vi "1lab11111.vi"() -> ()   [LabVIEW 2020]
panel:
  out "погрешность,%":dbl
  in  "шаг t":dbl
  out "Q":dbl(graph)
  in  "C эталонное":dbl
  out "Meter":dbl(knob) scale=0.0..10.0
  out "I":dbl(graph)
  out "U":dbl(graph)
  out "C. мкФ":dbl
  out "Величина заряда, мКл":dbl
  out "t разрядки":dbl
  in  "U конечное":dbl
  in  "U":dbl
  in  "R":dbl
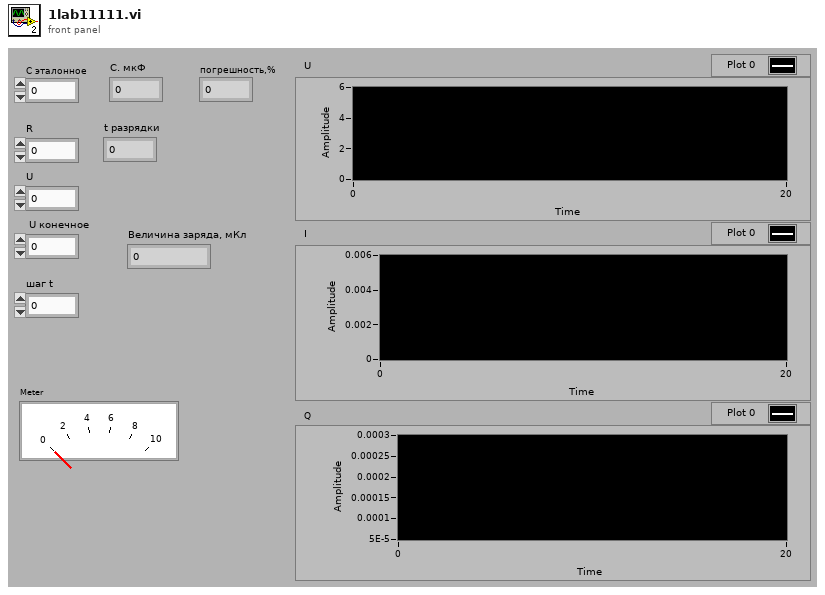
[diagram p1: front panel]
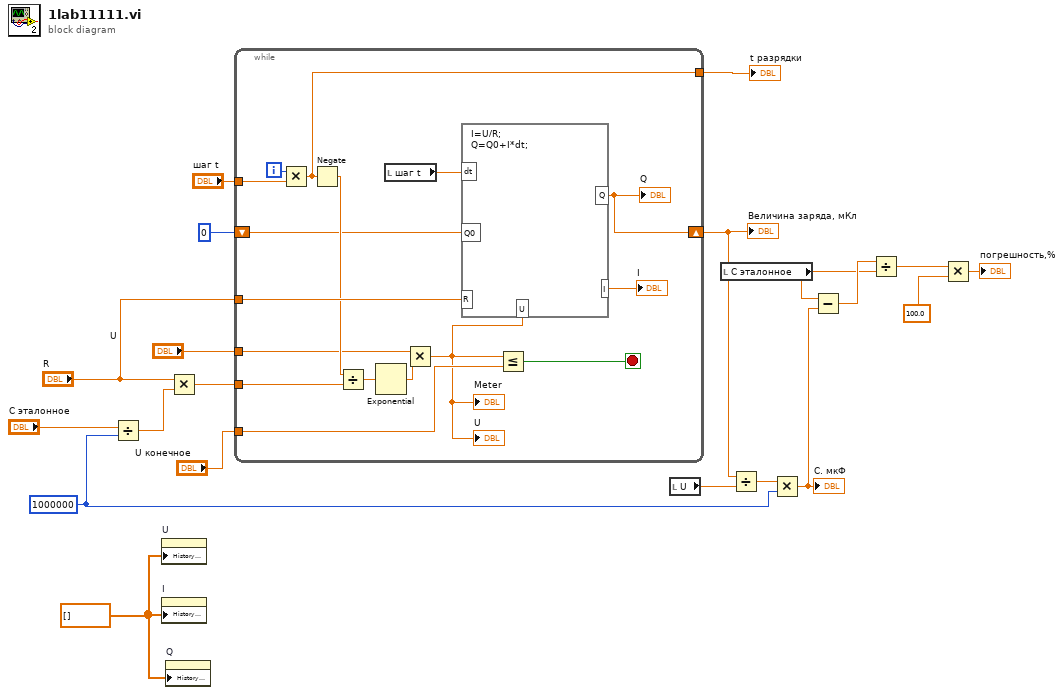
[diagram p0: block diagram]
diagram:
  w1 = dbl[] [] ("History Data")
  w15 = 1000000
  n1 = Divide(x="C эталонное", y=w15) -> (x/y=w19:dbl)
  n2 = property on="U" class="WFChart (strict)"("History Data"=w1) -> ()  [unwired: 2 in, 2 out]
  n3 = property on="I" class="WFChart (strict)"("History Data"=w1) -> ()  [unwired: 2 in, 2 out]
  n4 = property on="Q" class="WFChart (strict)"("History Data"=w1) -> ()  [unwired: 2 in, 2 out]
  n5 = Multiply(x="R", y=w19) -> (x*y=w17:dbl)
  n6 = while {
    tunnel: "R" -> [w34]
    tunnel: "U конечное" -> [w33]
    tunnel: w17 -> [w31]
    tunnel: "U" -> [w26]
    shift-right: [w25] -> w12
    shift-left: 0 -> [w27]
    tunnel: "шаг t" -> [w24]
    tunnel: [w23] -> w9
    i -> [w28]
    stop <- w35 stop-if-true
    n7 = Multiply(x=w28, y=w24) -> (x*y=w23:dbl)
    n8 = Negate(x=w23) -> (-x=w32:dbl)
    n9 = Divide(x=w32, y=w31) -> (x/y=w30:dbl)
    n10 = Exponential(1:w30) -> (0:w29:dbl)
    n11 = local read "шаг t"() -> (w21:dbl)
    n12 = Multiply(x=w26, y=w29) -> (x*y=w22:dbl)
    "U" <- w22
    "Meter" <- w22
    n13 = formula code="I=U/R;\nQ=Q0+I*dt;"("Q0"=w27, "R"=w34, "U"=w22, "dt"=w21) -> ("I"=→"I":dbl, "Q"=w25:dbl)
    "Q" <- w25
    n14 = Less Or Equal?(x=w22, y=w33) -> (x <= y?=w35:bool)
  }
  "t разрядки" <- w9
  "Величина заряда, мКл" <- w12
  n15 = local read "U"() -> (w11:dbl)
  n16 = local read "C эталонное"() -> (w6:dbl)
  n17 = Divide(x=w12, y=w11) -> (x/y=w8:dbl)
  n18 = Multiply(x=w8, y=w15) -> (x*y=w2:dbl)
  "C. мкФ" <- w2
  n19 = Subtract(x=w6, y=w2) -> (x-y=w7:dbl)
  n20 = Divide(x=w7, y=w6) -> (x/y=w5:dbl)
  n21 = Multiply(x=w5, y=100.0) -> (x*y=→"погрешность,%":dbl)
